vi "lsl empty.vi"(8 "error in (no error)":errorcluster, 11 "e":cluster{}) -> (0 "error out":errorcluster, 2 "function return":i32, 3 "e out":cluster{})   [LabVIEW 2016, in "Lab Streaming Layer.lvlib"]
doc: "extern LIBLSL_C_API int32_t lsl_empty(lsl_xml_ptr e);"
uses:
  Lab Streaming Layer.lvlib
  <userlib>/liblsl-LabVIEW/liblsl64.dll
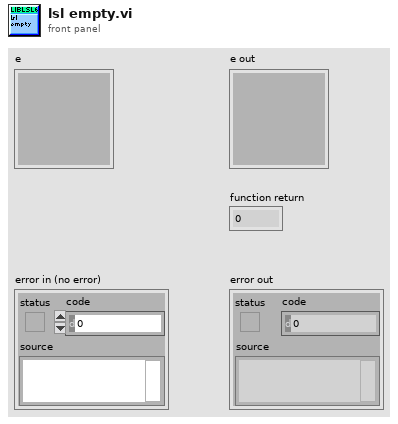
[diagram p1: front panel]
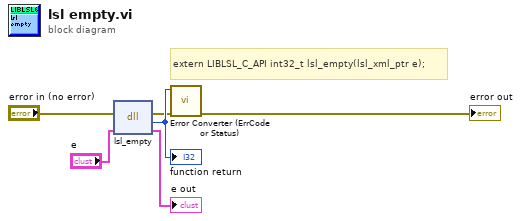
[diagram p0: block diagram]
diagram:
  # "extern LIBLSL_C_API int32_t lsl_empty(lsl_xml_ptr e);"
  n1 = dll-call lib="C:/Program Files/National Instruments/LabVIEW 2018/user.lib/liblsl-LabVIEW/liblsl64.*" fn="lsl_empty"(error in="error in (no error)", "e"="e") -> (error out=w2:errorcluster, w6:i32, "e"=→"e out":cluster{})  [unwired: 2 in, 1 out]
  "function return" <- w6
  n2 = call "Error Converter (ErrCode or Status).vi"("error in (no error)"=w2, "error code"=w6) -> ("error out"=→"error out":errorcluster)  [unwired: 9 in]
